vi "Override Transfers.vi"(8 "error in (no error)":errorcluster, 10 "Transfers":refnum<class "Transfer.lvclass">[](array[class]), 11 "Mock Transfer Group in":refnum<class "Mock Transfer Group.lvclass">) -> (0 "error out":errorcluster, 3 "Mock Transfer Group out":refnum<class "Mock Transfer Group.lvclass">)   [LabVIEW 2017, in "Mock Transfer Group.lvclass"]
uses:
  Mock Transfer Group.lvclass
  C:/github/data-sharing-framework/Data Sharing Framework Core/Engine/Classes/Transfer Group/Transfer Group.lvclass
  Engine/Classes/Transfer/Transfer.lvclass
  Engine/Classes/Transfer Group/Transfer Group.lvclass/Transfer Group.ctl
  Engine/Classes/Transfer Group/Transfer Group.lvclass
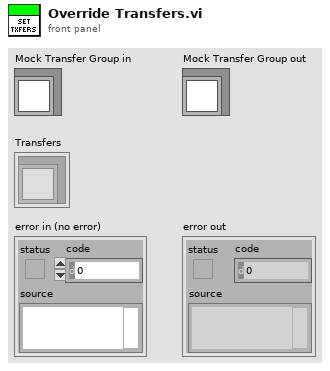
[diagram p1: front panel]
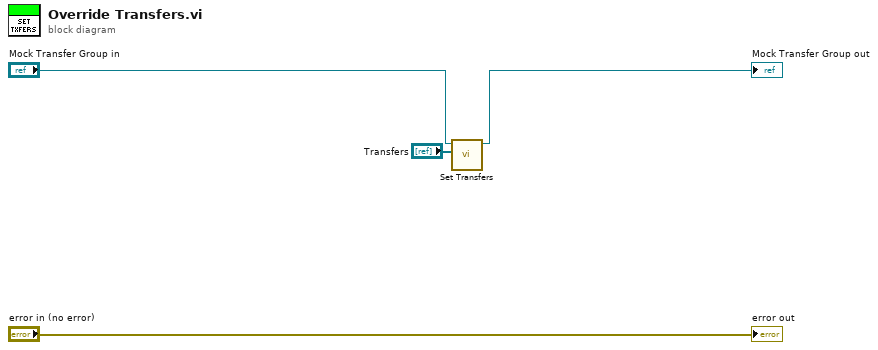
[diagram p0: block diagram]
diagram:
  n1 = call "Set Transfers.vi"("Transfers"="Transfers", "Transfer Group in"="Mock Transfer Group in") -> ("Transfer Group out"=→"Mock Transfer Group out":refnum<class "Mock Transfer Group.lvclass">)  [unwired: 9 in]
  "error out" <- "error in (no error)"
